vi "Date-Time string to DT format (2).vi"(1 "date/time string":string) -> (0 "Resulting Time Stamp":timestamp)   [LabVIEW 2010]
doc: "This VI convert a date/time string back to a time stamp."
panel:
  # "This control should have data in the form:\n4/30/2004 7:48:47 PM"
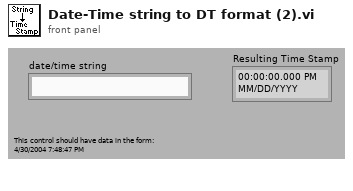
[diagram p1: front panel]
types:
  T1 = cluster{"second":i32, "minute":i32, "hour":i32, "day of month":i32, "month":i32, "year":i32, "day of week":i32, "day of year":i32, "is DST":i32}
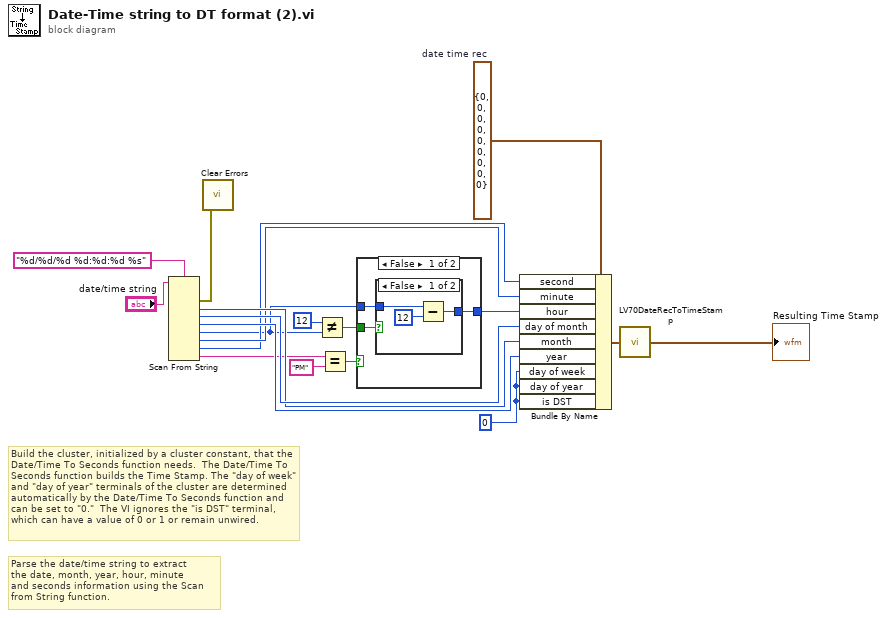
[diagram p0: block diagram]
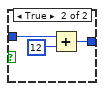
[diagram p4: hidden frame]
diagram:
  w1 = T1 {"second"=0, "minute"=0, "hour"=0, "day of month"=0, "month"=0, "year"=0, "day of week"=0, "day of year"=0, "is DST"=0}  # date time rec
  w16 = 0
  # "Build the cluster, initialized by a cluster constant, that the Date/Time To Seconds function needs.  The Date/Time To Seconds function builds the Time Stamp. The \"day of week\" and \"day of year\" terminals of the cluster are determined automatically by the Date/Time To Seconds function and can be set to \"0.\"  The VI ignores the \"is DST\" terminal, which can have a value of 0 or 1 or remain unwired."
  # "Parse the date/time string to extract \nthe date, month, year, hour, minute \nand seconds information using the Scan\nfrom String function."
  n1 = Scan From String "Scan From String"(format string="%d/%d/%d %d:%d:%d %s", input string="date/time string") -> (error out=w3:errorcluster, output 1=w14:i32, output 2=w15:i32, output 3=w13:i32, output 4=w7:i32, output 5=w12:i32, output 6=w11:i32, output 7=w10:string)  [unwired: 9 in, 2 out]
  n2 = call <vilib>:"Clear Errors.vi"("error in (no error)"=w3) -> ()  [unwired: 6 in, 1 out]
  n3 = Not Equal?(x=12 ("y"), y=w7) -> (x != y?=w4:bool)
  n4 = Equal?(x=w10, y="PM") -> (x = y?=w5:bool)
  n5 = case shown="False" w5 {
    tunnel: w7 -> [w22 w28]
    tunnel: [w20 w27] -> w6
    tunnel: w4 -> [w21 w29]
    frame False {
      n6 = case shown="False" w21 {
        tunnel: w22 -> [w25 w26]
        tunnel: [w23 w26] -> w20
        frame False {
          n7 = Subtract(x=w25, y=12) -> (x-y=w23:i32)
        }
        frame True {
        }
      }
    }
    frame True {
      n8 = case shown="False" w29 {
        tunnel: w28 -> [w30 w32]
        tunnel: [w30 w31] -> w27
        frame False {
        }
        frame True {
          n9 = Add(x=w32, y=12) -> (x+y=w31:i32)
        }
      }
    }
  }
  n10 = Bundle By Name(cluster=w1, "second"=w11, "minute"=w12, "hour"=w6, "day of month"=w15, "month"=w14, "year"=w13, "day of week"=w16, "day of year"=w16, "is DST"=w16) -> (w2:T1)
  n11 = call <vilib>:"LV70DateRecToTimeStamp.vi"("date time rec"=w2) -> ("Time Stamp"=→"Resulting Time Stamp":timestamp)
